vi "Construct.vi"(8 "error in (no error)":errorcluster, 11 "SEQ I64 in":refnum<class "SEQ I64.lvclass">) -> (0 "error out":errorcluster, 3 "SEQ I64 out":refnum<class "SEQ I64.lvclass">)   [LabVIEW 2024, in "SEQ I64.lvclass"]
uses:
  SEQ I64.lvclass
  SEQ I64.lvclass/SEQ I64.ctl
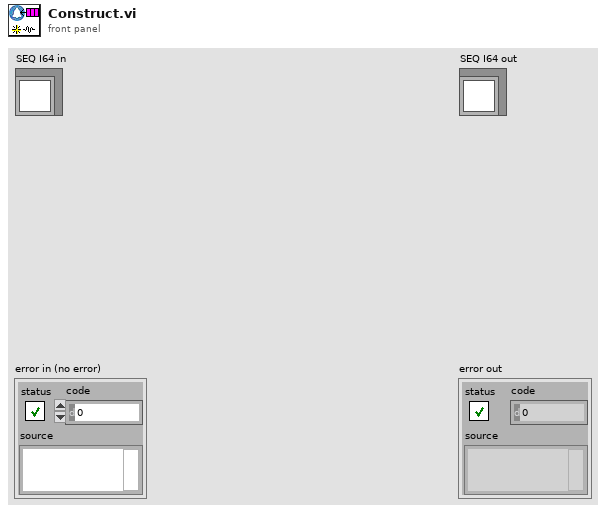
[diagram p1: front panel]
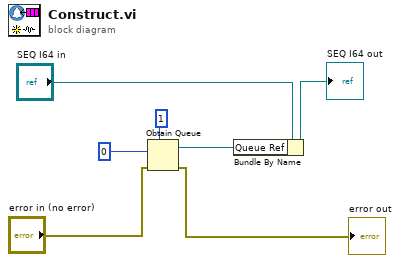
[diagram p0: block diagram]
diagram:
  n1 = Obtain Queue(max queue size (-1, unlimited)=1, element data type=i64 0, error in (no error)="error in (no error)") -> (queue out=w4:refnum<queue>, error out=→"error out":errorcluster)  [unwired: 2 in, 1 out]
  n2 = Bundle By Name(cluster="SEQ I64 in", "Queue Ref"=w4) -> (→"SEQ I64 out":refnum<class "SEQ I64.lvclass">)
